vi "Unix ns to Timestamp.vi"(3 "Unix ns":i64) -> (1 "Time Stamp":timestamp)   [LabVIEW 2020, in "Vecto.lvlib"]
uses:
  Vecto.lvlib
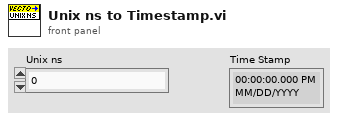
[diagram p1: front panel]
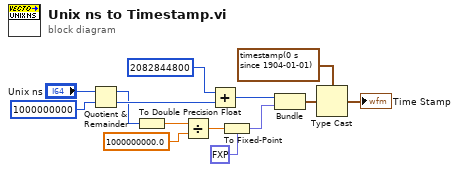
[diagram p0: block diagram]
diagram:
  n1 = Quotient & Remainder(x="Unix ns", y=i64 1000000000) -> (x-y*floor(x/y)=w6:i64, floor(x/y)=w7:i64)
  n2 = To Double Precision Float(number=w6) -> (double precision float=w5:dbl)
  n3 = Divide(x=w5, y=1000000000.0) -> (x/y=w3:dbl)
  n4 = Add(x=i64 2082844800 ("y"), y=w7) -> (x+y=w2:i64)
  n5 = To Fixed-Point(fixed-point type=fxp<+,64,0> 0.0, number=w3) -> (fixed-point=w12:fxp<+,64,0>)
  n6 = Bundle(w2, "fixed-point type"=w12) -> (w13:cluster{i64, "fixed-point type":fxp<+,64,0>})  [unwired: 1 in]
  n7 = Type Cast(type=timestamp(0 s since 1904-01-01) ("Time Stamp"), x=w13) -> (*(type *) &x=→"Time Stamp":timestamp)
